vi "8-bit video export-AVI close by mode.vi"(8 "error in (no error)":errorcluster, 11 "AVI modes refs":T1) -> (0 "error out":errorcluster, 3 "AVI modes refs":T1)   [LabVIEW 2017]
uses:
  Typedefs/8-bit video export AVI modes cluster.ctl
  <vilib>/vision/Avi1.llb/AviRefnum.ctl
  <vilib>/vision/Avi.llb/IMAQ AVI2 Refnum.ctl
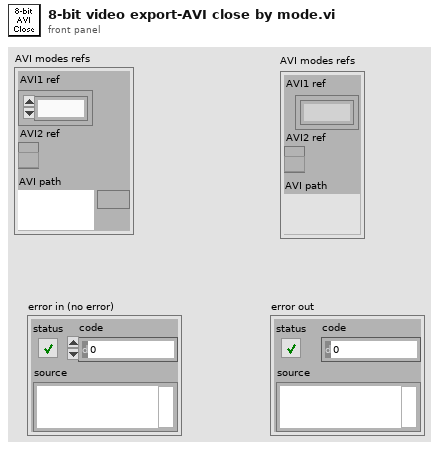
[diagram p1: front panel]
types:
  T1 = typedef "8-bit video export AVI modes cluster.ctl" = cluster{"AVI1 ref":T2, "AVI2 ref":T3, "AVI path":path}
  T2 = typedef "AviRefnum.ctl" = refnum<k1>
  T3 = typedef "IMAQ AVI2 Refnum.ctl" = refnum<k20>
  T4 = typedef "AVI implementation enum.ctl" = enum16{"AVI1", "AVI2"}
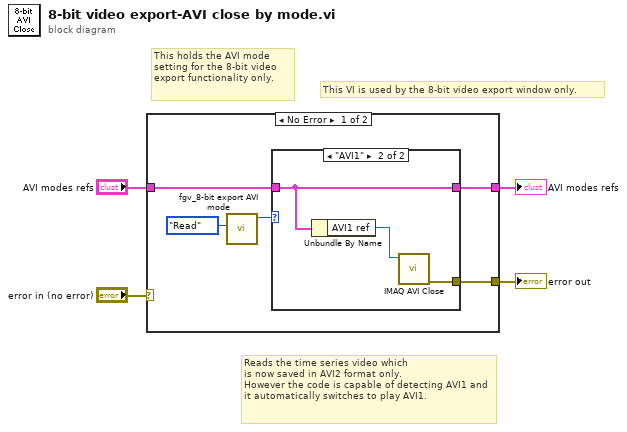
[diagram p0: block diagram]
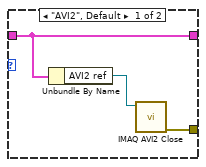
[diagram p2: hidden frame]
diagram:
  # "This VI is used by the 8-bit video export window only."
  # "This holds the AVI mode setting for the 8-bit video export functionality only."
  # "Reads the time series video which \nis now saved in AVI2 format only.\nHowever the code is capable of detecting AVI1 and it automatically switches to play AVI1."
  n1 = case shown="No Error" "error in (no error)" {
    selector: "error in (no error)" -> [_ w17]
    tunnel: "AVI modes refs" -> [w9 w16]
    tunnel: [w8 w16] -> w3
    tunnel: [w7 w17] -> w2
    frame No Error {
      n2 = call "fgv_8-bit export AVI mode.vi"("Function"=enum16{"Intialize", "Write", "Read", "Clear"}."Read") -> ("AVI mode"=w5:T4)  [unwired: 9 in, 1 out]
      n3 = case shown="\"AVI1\"" w5 {
        tunnel: [w12 w14] -> w7
        tunnel: w9 -> [w11 w15]
        tunnel: [w11 w15] -> w8
        frame "AVI2", Default {
          n4 = Unbundle By Name(w11) -> ("AVI2 ref"=w10:T3)
          n5 = call "IMAQ AVI2 Close"("AVI Refnum"=w10) -> ("error out"=w12:errorcluster)  [unwired: 10 in]
        }
        frame "AVI1" {
          n6 = Unbundle By Name(w15) -> ("AVI1 ref"=w13:T2)
          n7 = call "IMAQ AVI Close"("Avi Refnum"=w13) -> ("error out"=w14:errorcluster)  [unwired: 10 in]
        }
      }
    }
    frame Error {
    }
  }
  "error out" <- w2
  "AVI modes refs" <- w3
